vi "Update Clock.vi"(6 "timeout (ms)":i32=5000, 8 "error in (no error)":errorcluster, 10 "Clock Update":T1, 11 "CIFCorePlugin in":refnum<class "CIFCorePlugin.lvclass">) -> (0 "error out":errorcluster)   [LabVIEW 2021, in "CIFCorePlugin.lvclass"]
doc: "It registers an update of a time pair to track an external clock. \n \nThe ClockID can be read from the system and is set via gRPC for the plugin.\nSystem Time is the OS time. External time is the clock to be tracked. \nIf this is the first update or if external time has jumped (had a discontinuity, gone backwards, etc) then the reinit should be set true.\nThe clock name is used for tracking and logging.\n\nUpdates will be passed to the CIF manager on the system. Then the clock conversion will be updated and automatically passed to all plugins. \n\nThis VI makes a gRPC client call and will be non-deterministic. For time critical applications this should not be called in the time critical loop and instead the Update Clock Main.vi should be used."
uses:
  CIFCorePlugin.lvclass
  <vilib>/CIF Foundation/CIF Utilities/Time/Typedef/Clock Update.ctl
  <vilib>/CIF Foundation/CIF Utilities/Time/Typedef/Timestamp Pair.ctl
  CIFCorePlugin.lvclass/CIFCorePlugin.ctl
  CIFPluginManager/gRPC/CIF_Manager_Client_Wrapper/CIFManagerClientWrapper.lvlib
  <vilib>/CIF Foundation/CIF Utilities/Time/Time_CIF_U.lvlib
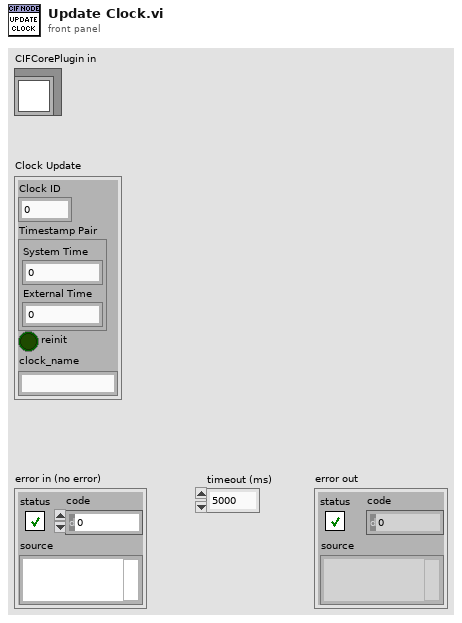
[diagram p1: front panel]
types:
  T1 = typedef "Time_CIF_U.lvlib/Clock Update.ctl" = cluster{"Clock ID":u8, "Timestamp Pair":T2, "reinit":bool, "clock_name":string}
  T2 = typedef "Time_CIF_U.lvlib/Timestamp Pair.ctl" = cluster{"System Time":i64, "External Time":i64}
  T3 = typedef "grpc-lvsupport-release.lvlib/grpcId.ctl" = u64
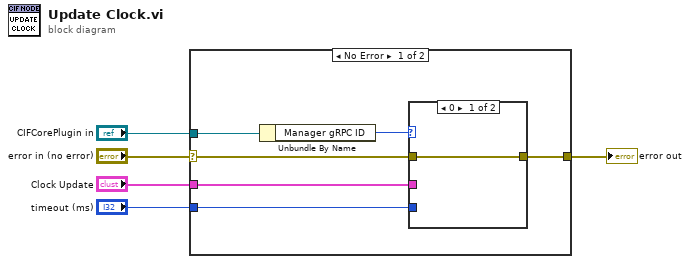
[diagram p0: block diagram]
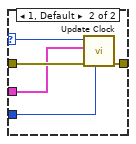
[diagram p2: hidden frame]
diagram:
  n1 = case shown="No Error" "error in (no error)" {
    selector: "error in (no error)" -> [w11 w18]
    tunnel: [w10 w18] -> w4
    tunnel: "CIFCorePlugin in" -> [w7 _]
    tunnel: "Clock Update" -> [w9 _]
    tunnel: "timeout (ms)" -> [w8 _]
    frame No Error {
      n2 = Unbundle By Name(w7) -> ("Manager gRPC ID"=w6:T3)
      n3 = case shown="0" w6 {
        selector: w6 -> [_ w13]
        tunnel: w11 -> [w12 w17]
        tunnel: [w12 w16] -> w10
        tunnel: w9 -> [_ w15]
        tunnel: w8 -> [_ w14]
        frame 0 {
        }
        frame 1, Default {
          n4 = call "Update Clock.vi"("timeout (ms)"=w14, "error in"=w17, "Clock Update"=w15, "gRPC ID in"=w13) -> ("error out"=w16:errorcluster)  [unwired: 6 in, 1 out]
        }
      }
    }
    frame Error {
    }
  }
  "error out" <- w4
